vi "Polynomial Normalization (DBL).vi"(1 "polynomial":dbl[](array[numeric])) -> (0 "normalized polynomial":dbl[](array[numeric]))   [LabVIEW 2017, in "NI_AALPro.lvlib"]
uses:
  NI_AALPro.lvlib
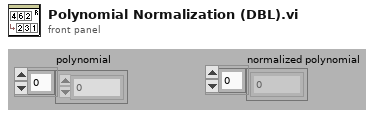
[diagram p1: front panel]
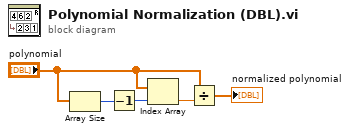
[diagram p0: block diagram]
diagram:
  n1 = Array Size(array="polynomial") -> (size(s)=w5:i32)
  n2 = Decrement(x=w5) -> (x-1=w4:i32)
  n3 = Index Array(array="polynomial", index=w4) -> (element=w3:dbl)
  n4 = Divide(x="polynomial", y=w3) -> (x/y=→"normalized polynomial":dbl[])
